vi "Async-Call with AdvanceAPI.vi"   [LabVIEW 2020]
uses:
  <userlib>/_NEVSTOP/JKI State Machine++/JKI State Machine++.lvlib
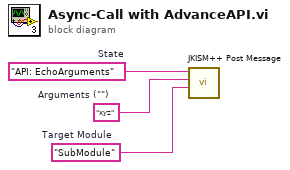
[diagram p0: block diagram]
diagram:
  w1 = "SubModule"  # Target Module
  w2 = "xyz"  # Arguments ("")
  w3 = "API: EchoArguments"  # State
  n1 = call <userlib>:"JKISM++ Post Message.vi"("Target Module"=w1, "Arguments (\"\")"=w2, "State"=w3) -> ()  [unwired: 8 in, 1 out]
